vi "ROI group-Extract group names from control array.vi"(1 "Groups":T1[](array[typedef])) -> (0 "Group Names Array":string[](array[string]))   [LabVIEW 2020]
uses:
  Typedefs/Group sel cluster.ctl
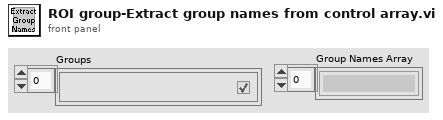
[diagram p1: front panel]
types:
  T1 = typedef "Group sel cluster.ctl" = cluster{"Group number":string, "Group Name":string, "Visibility":bool, "Highlight":bool}
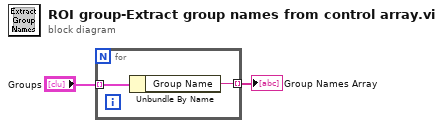
[diagram p0: block diagram]
diagram:
  n1 = for {
    tunnel: "Groups" -> [w4] mode=indexing
    tunnel: [w3] -> w2 mode=indexing
    n2 = Unbundle By Name(w4) -> ("Group Name"=w3:string)
  }
  "Group Names Array" <- w2
